vi "Validate.vi"(8 "error in":errorcluster, 10 "parameters":variant, 11 "Repository in":refnum<class "SystemConfigRepo.lvclass">) -> (0 "error out":errorcluster, 3 "Repository out":refnum<class "SystemConfigRepo.lvclass">)   [LabVIEW 2013, in "PL Framework Configuration Tool.lvlib" / "SystemConfigRepo.lvclass"]
doc: "An abstract method for validating the information inside of a repo is accurate. This method should be called before saving the information to file."
uses:
  SystemConfigRepo.lvclass
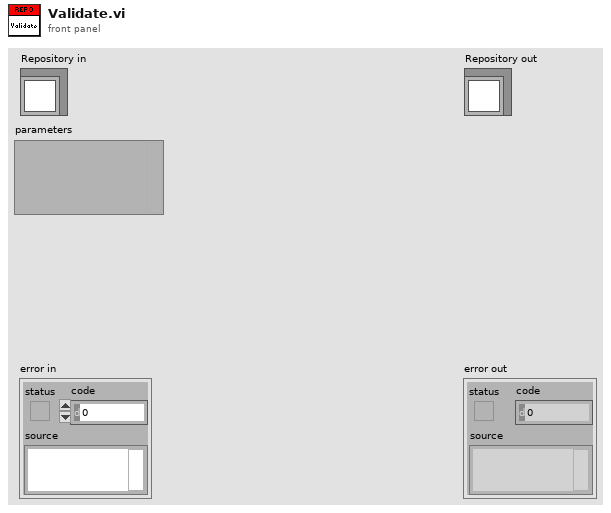
[diagram p1: front panel]
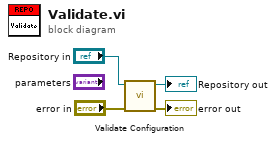
[diagram p0: block diagram]
diagram:
  n1 = call "Validate Configuration.vi"("error in"="error in", "SystemConfigRepo in"="Repository in") -> ("error out"=→"error out":errorcluster, "SystemConfigRepo out"=→"Repository out":refnum<class "SystemConfigRepo.lvclass">)  [unwired: 8 in]
